vi "Create Engine Folder and Copy RT Template.vi"(8 "error in (no error)":errorcluster, 9 "Project Root":path, 10 "Project Name":string, 11 "CD Template":refnum<class "NIVS_PPL_Inline HW Interface (Inline-Async).lvclass">) -> (0 "error out":errorcluster)   [LabVIEW 2019, in "NIVS_PPL_Inline HW Interface (Inline-Async).lvclass"]
uses:
  NIVS_PPL_Inline HW Interface (Inline-Async).lvclass
  NIVS_Consolidated_CDW_MetaDataObj/CD Engine lvlib.ctl
  NIVS_Consolidated_CDW_MetaDataObj/NIVS_Consolidated_CDW_MetaDataObj.lvclass
  NIVS_Consolidated_CDW_MetaDataObj/Common.ctl
  NIVS_Consolidated_CDW_MetaDataObj/CD Engine lvlib.vi
  NIVS_Consolidated_CDW_MetaDataObj/Common.vi
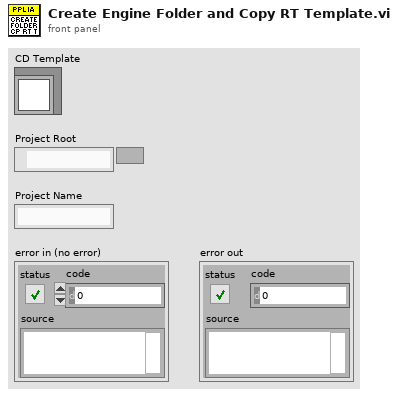
[diagram p1: front panel]
types:
  T1 = typedef "NIVS_Consolidated_CDW_MetaDataObj.lvclass/CD Engine lvlib.ctl" = enum16{"LibraryFileName", "LibraryFolderName", "Engine.FolderName", "Engine.Init.FolderName", "Engine.Run.FolderName", "Engine.Shutdown.FolderName", "Types.FolderName", "Engine.RT Driver VI.TemplatePath", "Engine.RT Driver VI.FileName", "Engine.PPL.RT Driver VI_InlineAsync.FileName", "Engine.RTStateVariables.Name", "Engine.PPL.RTStateVariables.Name", "Engine.RTStateVariables.Name.NoExtension", "Engine.Async.NameExtension", "Engine.Async.TemplateName", "Engine.PPL.Async.TemplateName", "Engine.PPL.Async.InitVSGlobals.Name"}
  T2 = typedef "NIVS_Consolidated_CDW_MetaDataObj.lvclass/Common.ctl" = enum16{"ProjectName", "TemplatesFolderName", "PPLTemplatesFolderName", "ProjectTemplatePathAndName", "ProjectPPLTemplatePathAndName", "TimingAndSyncFolderName", "CustomDeviceFolderName", "PathToTemplates", "PathToPPLTemplates", "PathToExplorerPPLTemplates", "PathToEnginePPLTemplates", "PathToConfigurationFile", "ProjectConfigurationName"}
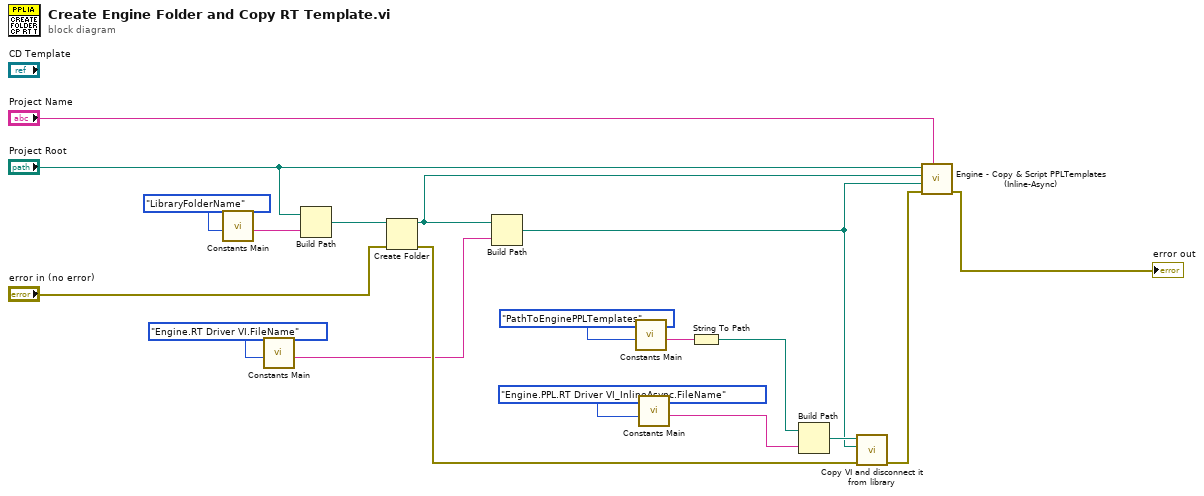
[diagram p0: block diagram]
diagram:
  n1 = call-poly "Constants Main.vi"("Action"=CD_Engine_lvlib."LibraryFolderName") -> ("Output"=w13:string)  [unwired: 10 in]
  n2 = call-poly "Constants Main.vi"("Action"=CD_Engine_lvlib."Engine.RT Driver VI.FileName") -> ("Output"=w17:string)  [unwired: 10 in]
  n3 = Build Path(base path="Project Root", name or relative path=w13) -> (appended path=w11:path)
  n4 = Create Folder(path (use dialog)=w11, error in="error in (no error)") -> (created path=w6:path, error out=w19:errorcluster)  [unwired: 1 in, 1 out]
  n5 = Build Path(base path=w6, name or relative path=w17) -> (appended path=w4:path)
  n6 = call-poly "Constants Main.vi"("Action"=Common."PathToEnginePPLTemplates") -> ("Output"=w16:string)  [unwired: 10 in]
  n7 = call-poly "Constants Main.vi"("Action"=CD_Engine_lvlib."Engine.PPL.RT Driver VI_InlineAsync.FileName") -> ("Output"=w2:string)  [unwired: 10 in]
  n8 = String To Path(string=w16) -> (path=w9:path)
  n9 = Build Path(base path=w9, name or relative path=w2) -> (appended path=w15:path)
  n10 = call "Copy VI and disconnect it from library.vi"("error in (no error)"=w19, "VI Target Path"=w4, "VI Source Path"=w15) -> ("error out"=w3:errorcluster)  [unwired: 8 in]
  n11 = call "Engine - Copy & Script PPLTemplates (Inline-Async).vi"("CD Name"="Project Name", "error in (no error)"=w3, "RT Driver VI Path"=w4, "RT Driver Folder Path"=w6, "CD Source Folder Path"="Project Root") -> ("error out"=→"error out":errorcluster)  [unwired: 6 in]
